vi "Even Sigma.vi"() -> ()   [LabVIEW 2016]
uses:
  <vilib>/express/express arith-compare/Formula/XNode/ExpressFormulaBlockNode.xnode
panel:
  out "OP":dbl
  in  "Y end":dbl
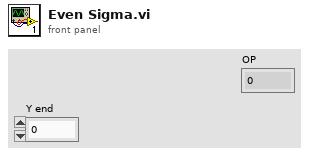
[diagram p1: front panel]
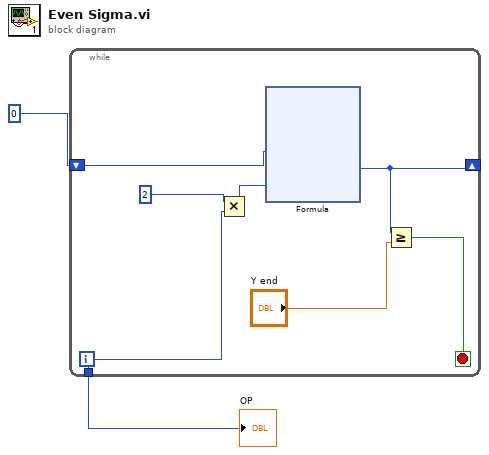
[diagram p0: block diagram]
diagram:
  n1 = while {
    shift-right: [w5] -> _
    shift-left: 0 -> [w7]
    tunnel: [w6] -> w1
    i -> [w6]
    stop <- w3 stop-if-true
    n2 = Multiply(x=2, y=w6) -> (x*y=w8:i32)
    n3 = xnode "Formula"("A"=w7, "B"=w8) -> ("Result"=w5:i32)  [unwired: 1 in, 1 out]
    n4 = Greater Or Equal?(x=w5, y="Y end") -> (x >= y?=w3:bool)
  }
  "OP" <- w1
